vi "PathPlanner_PathPoint_Flip.vi"(11 "PathPlannerPoint":T1={"Position"={"X"=0.0, "Y"=0.0}, "DistAlongPath"=0.0, "MaxV"=9e+300, "Constraints"={"MaxVelocityMps;"=0.0, "MaxAccelerationMpsSq;"=0.0, "MaxAngularVelRadPsEc;"=0.0, "MaxAngularAccRadPSecSq"=0.0, "Exists"=FALSE, "Unlimited"=FALSE, "NominalVoltageVolts"=12.0}, "RotationTarget"={"position"=1.0, "rotation"={"VALUE"=0.0, "COS"=0.0, "SIN"=0.0}, "Exists"=FALSE}, "WaypointRelativePos"=0.0} {"RotationTarget"."rotation"."SIN" format="%13.4f"; "RotationTarget"."rotation"."COS" format="%13.4f"; "RotationTarget"."rotation"."VALUE" format="%13.4f"; "Position"."Y" format="%14.3f"; "Position"."X" format="%14.3f"}) -> (3 "FlippedPathPlannerPoint":T1={"Position"={"X"=0.0, "Y"=0.0}, "DistAlongPath"=0.0, "MaxV"=9e+300, "Constraints"={"MaxVelocityMps;"=0.0, "MaxAccelerationMpsSq;"=0.0, "MaxAngularVelRadPsEc;"=0.0, "MaxAngularAccRadPSecSq"=0.0, "Exists"=FALSE, "Unlimited"=FALSE, "NominalVoltageVolts"=12.0}, "RotationTarget"={"position"=1.0, "rotation"={"VALUE"=0.0, "COS"=0.0, "SIN"=0.0}, "Exists"=FALSE}, "WaypointRelativePos"=0.0} {"RotationTarget"."rotation"."SIN" format="%13.4f"; "RotationTarget"."rotation"."COS" format="%13.4f"; "RotationTarget"."rotation"."VALUE" format="%13.4f"; "Position"."Y" format="%14.3f"; "Position"."X" format="%14.3f"})   [LabVIEW 2019, in "PathPlanner24.lvlib"]
doc: "Flip this path point to the other side of the field, maintaining a blue alliance origin\n\nInputs:\n -- PathPoint - cluster - point definition\n\nOutputs:\n -- FlippedPathPoint - cluster - flipped point definition"
uses:
  PathPlanner24.lvlib
  TypeDef/PathPlannerPathPoint.ctl
  <vilib>/Rock Robotics/WPI/ThirdParty/JAS_Junk/TrajLib/TypeDef/TRANSLATION2D.ctl
  TypeDef/PathPlannerPathConstraints.ctl
  TypeDef/PathPlannerRotationTarget.ctl
  <vilib>/Rock Robotics/WPI/ThirdParty/JAS_Junk/TrajLib/TypeDef/ROTATION2D.ctl
  PathPlanner_RotationTarget_New.vi
  PathPlanner_RotationTarget_GetAll.vi
  PathPlanner_FieldUtil_FlipFieldRotation.vi
  PathPlanner_FieldUtil_SymmetryType.vi
  PathPlanner_FieldUtil_FieldSizeY.vi
  <vilib>/Rock Robotics/WPI/ThirdParty/JAS_Junk/TrajLib/Translation2d_GetXY.vi
  <vilib>/Rock Robotics/WPI/ThirdParty/JAS_Junk/TrajLib/Translation2d_Create.vi
  PathPlanner_FieldUtil_FieldSizeX.vi
  <vilib>/Rock Robotics/WPI/ThirdParty/JAS_Junk/TrajLib/Rotation2d_CreateAngle.vi
  <vilib>/Rock Robotics/WPI/ThirdParty/JAS_Junk/TrajLib/Rotation2d_Minus.vi
  <vilib>/Rock Robotics/WPI/ThirdParty/JAS_Junk/TrajLib/Conv_Feet_Meters.vi
  <vilib>/Rock Robotics/WPI/ThirdParty/JAS_Junk/TrajLib/Rotation2d_UnaryMinus.vi
  <vilib>/Rock Robotics/WPI/ThirdParty/JAS_Junk/TrajLib/Rotation2d_RotateBy.vi
  <vilib>/Rock Robotics/WPI/ThirdParty/JAS_Junk/TrajLib/Rotation2d_CreateXY.vi
  <vilib>/Rock Robotics/WPI/ThirdParty/JAS_Junk/TrajLib/Util_CalcDist.vi
  <vilib>/Rock Robotics/WPI/ThirdParty/JAS_Junk/TrajLib/Trajectory_Library.lvlib
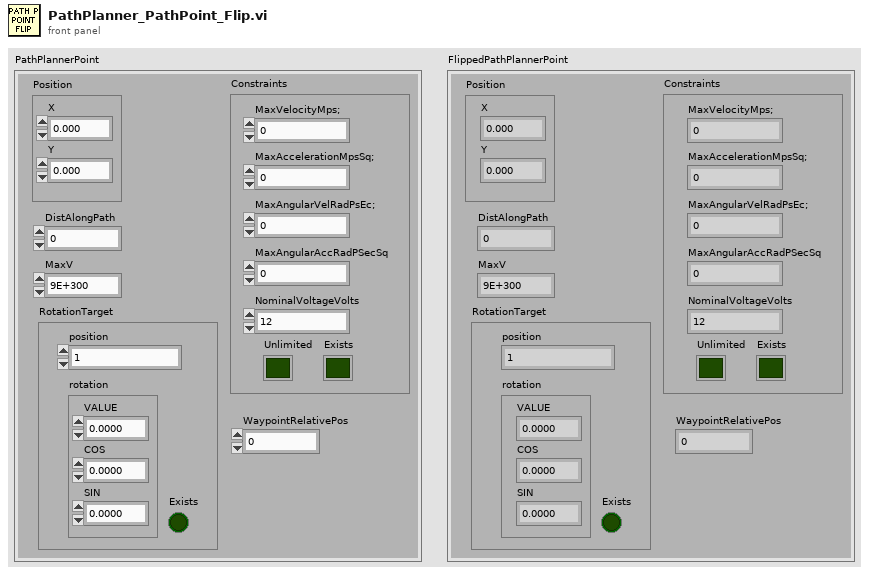
[diagram p1: front panel]
types:
  T1 = typedef "PathPlanner24.lvlib/PathPlannerPathPoint.ctl" = cluster{"Position":T2, "DistAlongPath":dbl, "MaxV":dbl, "Constraints":T3, "RotationTarget":T4, "WaypointRelativePos":dbl}
  T2 = typedef "Trajectory_Library.lvlib/TRANSLATION2D.ctl" = cluster{"X":dbl, "Y":dbl}
  T3 = typedef "PathPlanner24.lvlib/PathPlannerPathConstraints.ctl" = cluster{"MaxVelocityMps;":dbl, "MaxAccelerationMpsSq;":dbl, "MaxAngularVelRadPsEc;":dbl, "MaxAngularAccRadPSecSq":dbl, "Exists":bool, "Unlimited":bool, "NominalVoltageVolts":dbl}
  T4 = typedef "PathPlanner24.lvlib/PathPlannerRotationTarget.ctl" = cluster{"position":dbl, "rotation":T5, "Exists":bool}
  T5 = typedef "Trajectory_Library.lvlib/ROTATION2D.ctl" = cluster{"VALUE":dbl, "COS":dbl, "SIN":dbl}
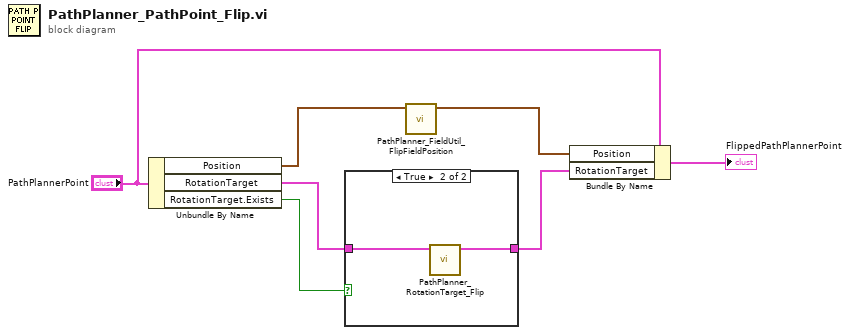
[diagram p0: block diagram]
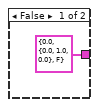
[diagram p2: hidden frame]
diagram:
  n1 = Unbundle By Name("PathPlannerPoint") -> ("Position"=w2:T2, "RotationTarget"=w4:T4, "RotationTarget.Exists"=w5:bool)
  n2 = case shown="True" w5 {
    tunnel: w4 -> [_ w10]
    tunnel: [T4 {"position"=0.0, "rotation"={"VALUE"=0.0, "COS"=1.0, "SIN"=0.0}, "Exists"=FALSE} ("FlippedRotationTarget") w9] -> w3
    frame False {
    }
    frame True {
      n3 = call "PathPlanner_RotationTarget_Flip.vi"("RotationTarget"=w10) -> ("FlippedRotationTarget"=w9:T4)  [unwired: 10 in]
    }
  }
  n4 = call "PathPlanner_FieldUtil_FlipFieldPosition.vi"("FieldPosition"=w2) -> ("FlippedFieldPosition"=w1:T2)  [unwired: 10 in]
  n5 = Bundle By Name(cluster="PathPlannerPoint", "Position"=w1, "RotationTarget"=w3) -> (→"FlippedPathPlannerPoint":T1)
